vi "Tegam4040 - DAC - Reader.vi"() -> ()   [LabVIEW 2010, in "Tegam4040.lvlib"]
uses:
  Tegam4040.lvlib
panel:
  out "value":u32 format="%x"
  in  "VISA Tegam4040":refnum<visa-resource-name>
  in  "error in (no error)":errorcluster
  out "VISA Out":refnum<visa-resource-name>
  out "error out":errorcluster
  in  "DAC":u16 format="%x"
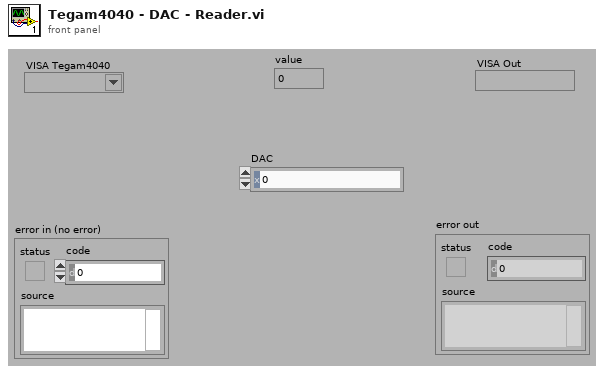
[diagram p1: front panel]
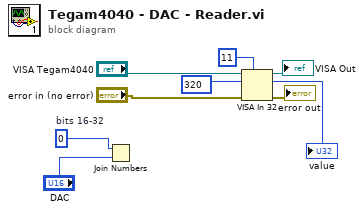
[diagram p0: block diagram]
diagram:
  w9 = u16 0  # bits 16-32
  n1 = Join Numbers(hi=w9, lo="DAC") -> ()  [unwired: 1 out]
  n2 = VISA In 32(7:u16 11 ("address space (A16:  1)"), 8:"error in (no error)", 10:u32 320 ("offset (0)"), 11:"VISA Tegam4040") -> (0:→"error out":errorcluster, 2:→"value":u32, 3:→"VISA Out":refnum<visa-resource-name>)
